vi "Drive Straight.vi"(11 "Distance to travel":dbl) -> (3 "In Range?":bool)   [LabVIEW 2015]
uses:
  Robot Values.vi
  <vilib>/addons/control/pid/pid.llb/PID (DBL).vi
  Vision Target Values.vi
  <vilib>/addons/control/pid/NI_PID_pid.lvlib
panel:
  in  "Tolerance":dbl=0.01
  in  "PID Error Gains":T1={"proportional gain (Kc)"=1.0, "integral time (Ti, min)"=0.01, "derivative time (Td, min)"=0.0} {"derivative time (Td, min)" format="%.3f"; "integral time (Ti, min)" format="%.3f"; "proportional gain (Kc)" format="%.3f"}
  in  "PID gains":T1={"proportional gain (Kc)"=1.0, "integral time (Ti, min)"=0.01, "derivative time (Td, min)"=0.0} {"derivative time (Td, min)" format="%.3f"; "integral time (Ti, min)" format="%.3f"; "proportional gain (Kc)" format="%.3f"}
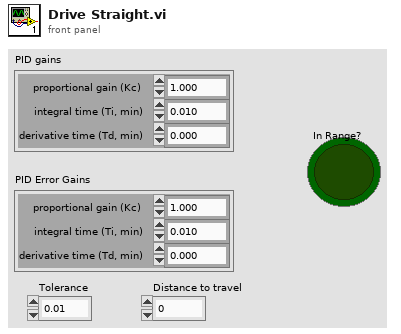
[diagram p1: front panel]
types:
  T1 = cluster{"proportional gain (Kc)":dbl, "integral time (Ti, min)":dbl, "derivative time (Td, min)":dbl}
  T2 = cluster{"Detected Targets":cluster{"Distance (ft)":dbl, "Center":cluster{"X":dbl, "Y":dbl}, "Normalized Rect":cluster{"Numeric":dbl, "Numeric 2":dbl, "Numeric 3":dbl, "Numeric 5":dbl}}[]}
  T3 = typedef "Robot Values.ctl" = cluster{"Drive Motors":cluster{"Left Motor Value":dbl, "Right Motor Value":dbl, "Left Motor Encoder":dbl, "Right Motor Encoder":dbl, "High/Low Gear":bool}, "Sensors":cluster{"Gyro Angle":dbl, "Photoeye":bool, "Ultrasonic Range":dbl, "Shooter Speed Encoder":dbl, "Accelerometer Value":dbl, "Flashlight":bool}, "Arms":cluster{"Desired Arm Position":dbl, "Left Arm Encoder":dbl, "Right Arm Encoder":dbl, "Left Arm Lower Limit":bool, "Right Arm Lower Limit":bool}, "Acquisition and Scoring":cluster{"Acquiring?":bool, "Current Speed":dbl, "Setpoint Speed":dbl, "Prep Wheels":bool, "Shoot":bool, "Low Eject":bool}, "Hanging":cluster{"Pivot Arms":dbl, "PTO":bool, "Left Erector":dbl, "Right Erector":dbl, "Hanging Pin":bool}}
  T4 = cluster{"Distance (ft)":dbl, "Center":cluster{"X":dbl, "Y":dbl}, "Normalized Rect":cluster{"Numeric":dbl, "Numeric 2":dbl, "Numeric 3":dbl, "Numeric 5":dbl}}[]
  T5 = cluster{"Distance (ft)":dbl, "Center":cluster{"X":dbl, "Y":dbl}, "Normalized Rect":cluster{"Numeric":dbl, "Numeric 2":dbl, "Numeric 3":dbl, "Numeric 5":dbl}}
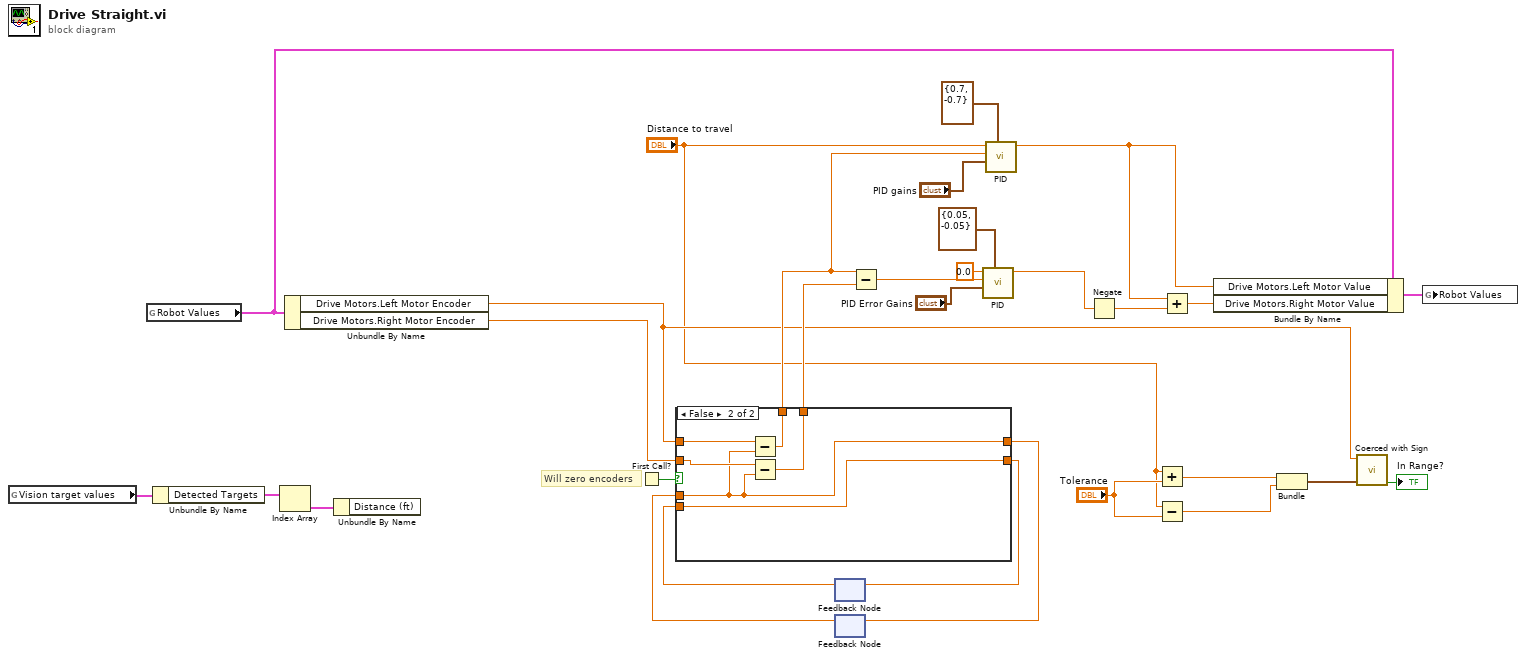
[diagram p0: block diagram]
diagram:
  # "Will zero encoders"
  n1 = global read "Vision Target Values.vi" "Vision target values"() -> (w3:T2)
  n2 = global read "Robot Values.vi" "Robot Values"() -> (w16:T3)
  n3 = Unbundle By Name(w3) -> ("Detected Targets"=w2:T4)
  n4 = Index Array(array=w2) -> (element=w1:T5)  [unwired: 1 in]
  n5 = Unbundle By Name(w16) -> ("Drive Motors.Left Motor Encoder"=w11:dbl, "Drive Motors.Right Motor Encoder"=w25:dbl)
  n6 = Unbundle By Name(w1) -> ()  [unwired: 1 out]
  n7 = First Call?() -> (First Call?: T/F=w4:bool)
  n8 = feedback #1() -> (w22:dbl)  [unwired: 1 in]
  n9 = feedback #2() -> (w21:dbl)  [unwired: 1 in]
  n10 = case shown="False" w4 {
    tunnel: w11 -> [w32 w37]
    tunnel: w25 -> [w31 w36]
    tunnel: [w32 w35] -> w23
    tunnel: [w31 w38] -> w24
    tunnel: w22 -> [_ w38]
    tunnel: w21 -> [_ w35]
    tunnel: [_ w34] -> w20
    tunnel: [_ w33] -> w19
    frame True {
    }
    frame False {
      n11 = Subtract(x=w37, y=w35) -> (x-y=w33:dbl)
      n12 = Subtract(x=w36, y=w35) -> (x-y=w34:dbl)
    }
  }
  n13 = feedback-in #1(w24) -> ()
  n14 = feedback-in #2(w23) -> ()
  n15 = Subtract(x=w19, y=w20) -> (x-y=w28:dbl)
  n16 = call-poly <vilib>:"PID.vi"("output range"=cluster{"output high":dbl, "output low":dbl} {"output high"=0.05, "output low"=-0.05}, "PID gains"="PID Error Gains", "process variable"=w28, "setpoint"=0.0) -> ("output"=w13:dbl)  [unwired: 6 in, 1 out]
  n17 = call-poly <vilib>:"PID.vi"("output range"=cluster{"output high":dbl, "output low":dbl} {"output high"=0.7, "output low"=-0.7}, "PID gains"="PID gains", "process variable"=w19, "setpoint"="Distance to travel") -> ("output"=w14:dbl)  [unwired: 6 in, 1 out]
  n18 = Negate(x=w13) -> (-x=w12:dbl)
  n19 = Add(x="Distance to travel", y="Tolerance") -> (x+y=w6:dbl)
  n20 = Subtract(x="Distance to travel", y="Tolerance") -> (x-y=w7:dbl)
  n21 = Add(x=w14, y=w12) -> (x+y=w15:dbl)
  n22 = Bundle By Name(cluster=w16, "Drive Motors.Left Motor Value"=w14, "Drive Motors.Right Motor Value"=w15) -> (w17:T3)
  n23 = Bundle(w6, w7) -> (w5:cluster{dbl, dbl})  [unwired: 1 in]
  n24 = call "Coerced with Sign.vi"("Input"=w11, "Limits"=w5) -> ("In Range?"=→"In Range?":bool)  [unwired: 7 in, 1 out]
  n25 = global write "Robot Values.vi" "Robot Values"(w17) -> ()
